vi "低层函数-连续.vi"() -> ()   [LabVIEW 2018]
uses:
  <vilib>/userdefined/High Color/IMAQdx.ctl
  <vilib>/vision/driver/IMAQdx.llb/IMAQdx Acquisition Mode.ctl
  <vilib>/vision/driver/IMAQdx.llb/IMAQdx Buffer Number Mode.ctl
  <vilib>/vision/driver/NI_Vision_Acquisition_Software.lvlib
panel:
  in  "布尔":bool
  out "error out":errorcluster
  out "Buffer Number Out":u32
  out "Image":T1(plugin-control)
  in  "error in":errorcluster
  in  "Session In":T2
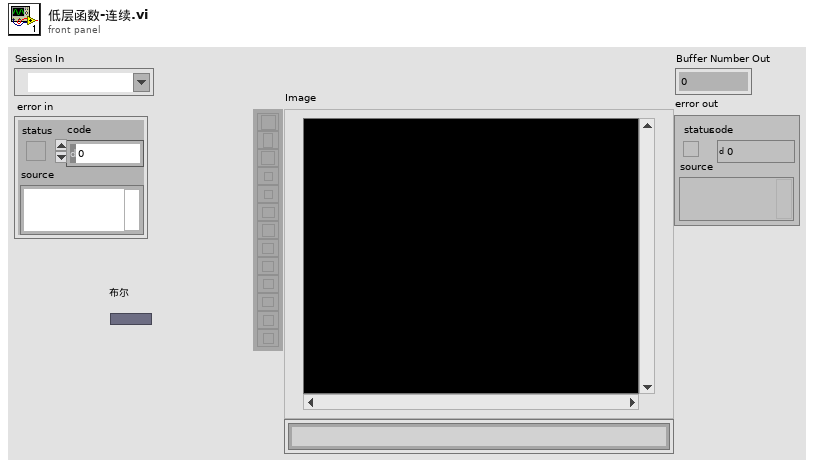
[diagram p1: front panel]
types:
  T1 = typedef "IMAQ Image.ctl" = refnum<image>
  T2 = typedef "IMAQdx.ctl" = refnum<k21>
  T3 = typedef "NI_Vision_Acquisition_Software.lvlib/IMAQdx Acquisition Mode.ctl" = enum32{"One Shot", "Continuous"}
  T4 = typedef "NI_Vision_Acquisition_Software.lvlib/IMAQdx Buffer Number Mode.ctl" = enum32{"Next", "Last", "Buffer Number", "Every", "Last New"}
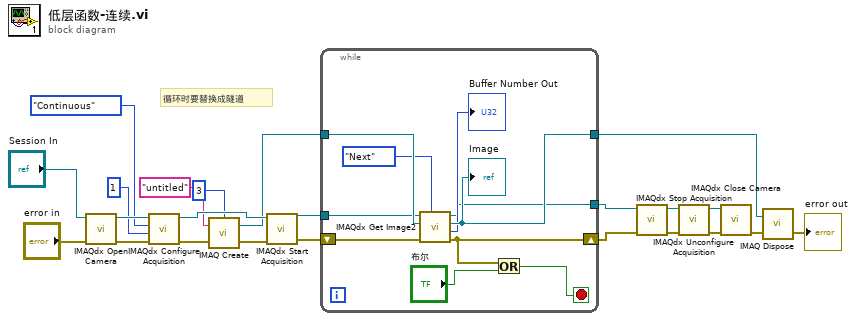
[diagram p0: block diagram]
diagram:
  # "循环时要替换成隧道"
  n1 = call <vilib>:"IMAQdx Open Camera.vi"("error in"="error in", "Session In"="Session In") -> ("error out"=w18:errorcluster, "Session Out"=w22:T2)  [unwired: 8 in]
  n2 = call <vilib>:"IMAQdx Configure Acquisition.vi"("error in"=w18, "Number of Buffers"=u32 1, "Continuous?"=IMAQdx_Acquisition_Mode."Continuous", "Session In"=w22) -> ("error out"=w23:errorcluster, "Session Out"=w17:T2)  [unwired: 6 in]
  n3 = call "IMAQ Create"("Border Size"=3, "Image Name"="untitled", "error in (no error)"=w23) -> ("New Image"=w15:T1, "error out"=w14:errorcluster)  [unwired: 2 in]
  n4 = call <vilib>:"IMAQdx Start Acquisition.vi"("error in"=w14, "Session In"=w17) -> ("error out"=w7:errorcluster, "Session Out"=w8:T2)  [unwired: 8 in]
  n5 = while {
    tunnel: w8 -> [w24]
    tunnel: [w28] -> w5
    shift-right: [w26] -> w6
    shift-left: w7 -> [w31]
    tunnel: w15 -> [w33]
    tunnel: [w32] -> w11
    stop <- w25 stop-if-true
    n6 = call <vilib>:"IMAQdx Get Image2.vi"("Buffer Number Mode (Next)"=IMAQdx_Buffer_Number_Mode."Next", "error in"=w31, "Image In"=w33, "Session In"=w24) -> ("error out"=w26:errorcluster, "Buffer Number Out"=→"Buffer Number Out":u32, "Image Out"=w32:T1, "Session Out"=w28:T2)  [unwired: 4 in]
    "Image" <- w32
    n7 = Or(x=w26, y="布尔") -> (x .or. y?=w25:bool)
  }
  n8 = call <vilib>:"IMAQdx Stop Acquisition.vi"("error in"=w6, "Session In"=w5) -> ("error out"=w3:errorcluster, "Session Out"=w4:T2)  [unwired: 8 in]
  n9 = call <vilib>:"IMAQdx Unconfigure Acquisition.vi"("error in"=w3, "Session In"=w4) -> ("error out"=w1:errorcluster, "Session Out"=w2:T2)  [unwired: 8 in]
  n10 = call <vilib>:"IMAQdx Close Camera.vi"("error in"=w1, "Session In"=w2) -> ("error out"=w12:errorcluster)  [unwired: 9 in]
  n11 = call "IMAQ Dispose"("Image"=w11, "error in (no error)"=w12) -> ("error out"=→"error out":errorcluster)  [unwired: 4 in]
